vi "Test_save log.vi"(8 "error in (no error)":errorcluster, 11 "Test":T1) -> (3 "Report":string)   [LabVIEW 2015]
uses:
  controls/Test Data.ctl
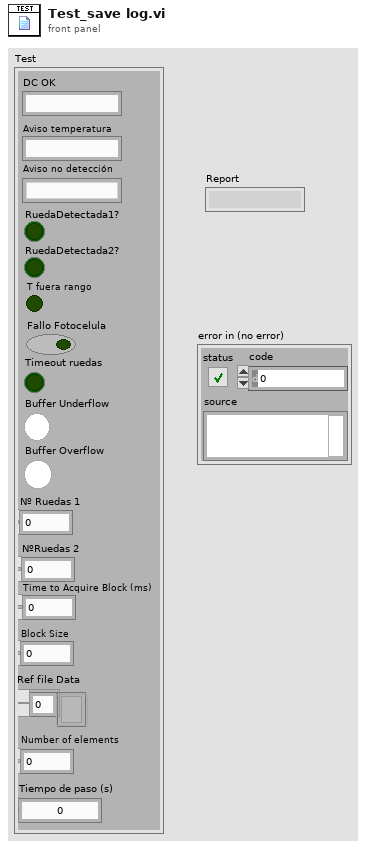
[diagram p1: front panel]
types:
  T1 = typedef "Test Data.ctl" = cluster{"DC OK":string, "Aviso temperatura":string, "Aviso no detección":string, "RuedaDetectada1?":bool, "RuedaDetectada2?":bool, "T fuera rango":bool, "Fallo Fotocelula":bool, "Timeout ruedas":bool, "Buffer Underflow":bool, "Buffer Overflow":bool, "Nº Ruedas 1":i32, "NºRuedas 2":i32, "Block Size":u32, "Time to Acquire Block (ms)":i32, "Ref file Data":refnum<file>[], "Number of elements":u32, "Tiempo de paso (s)":dbl}
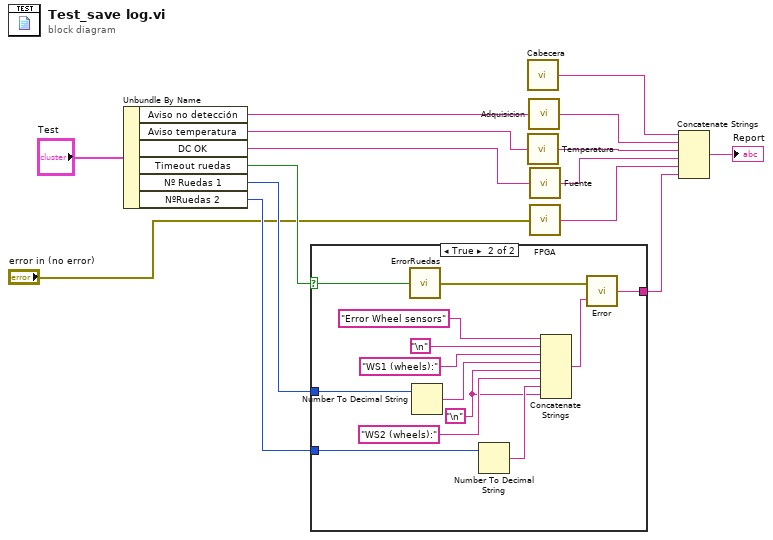
[diagram p0: block diagram]
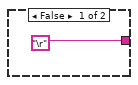
[diagram p2: hidden frame]
diagram:
  n1 = Unbundle By Name("Test") -> ("Aviso no detección"=w2:string, "Aviso temperatura"=w3:string, "DC OK"=w4:string, "Timeout ruedas"=w6:bool, "Nº Ruedas 1"=w12:i32, "NºRuedas 2"=w13:i32)
  n2 = case shown="True" w6 {
    selector: w6 -> [_ w27]
    tunnel: ["\r" w28] -> w14
    tunnel: w12 -> [_ w18]
    tunnel: w13 -> [_ w17]
    frame False {
    }
    frame True {
      w19 = "\n"
      n3 = call "ErrorRuedas.vi"("Buffer Overflow"=w27) -> ("error out"=w29:errorcluster)
      n4 = Number To Decimal String(number=w18) -> (decimal integer string=w23:string)  [unwired: 1 in]
      n5 = Number To Decimal String(number=w17) -> (decimal integer string=w20:string)  [unwired: 1 in]
      n6 = Concatenate Strings("Error Wheel sensors", "\n", "WS1 (wheels):", w23, w19, "WS2 (wheels):", w20, w19) -> (w21:string)
      n7 = call "Error.vi"("Error con..."=w21, "error comunicacion 2"=w29) -> ("String"=w28:string)
    }
  }
  n8 = call "Cabecera.vi"() -> ("String"=w7:string)
  n9 = call "Temperatura.vi"("Aviso temperatura"=w3) -> ("String"=w9:string)
  n10 = call "Adquisicion.vi"("Aviso no detección"=w2) -> ("String"=w8:string)
  n11 = call "Fuente.vi"("DC OK"=w4) -> ("String"=w10:string)
  n12 = call "FPGA.vi"("error out"="error in (no error)") -> ("String"=w11:string)
  n13 = Concatenate Strings(w7, w8, w9, w10, w11, w14) -> (→"Report":string)
